vi "L_Cal_XYZ_Coordinate.vi"(9 "distance":dbl, 10 "vertical":dbl, 11 "azimuth":dbl) -> (1 "z":dbl, 2 "y":dbl, 3 "x":dbl)   [LabVIEW 2019]
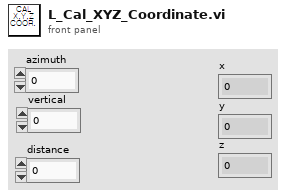
[diagram p1: front panel]
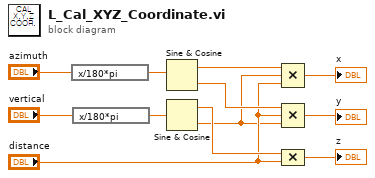
[diagram p0: block diagram]
diagram:
  n1 = expression code="x/180*pi"("azimuth") -> (w10:dbl)
  n2 = expression code="x/180*pi"("vertical") -> (w9:dbl)
  n3 = Sine & Cosine(0:w10) -> (1:w8:dbl, 2:w6:dbl)
  n4 = Sine & Cosine(0:w9) -> (1:w3:dbl, 2:w1:dbl)
  n5 = Compound Arithmetic op=MULTIPLY(w8, w1, "distance") -> (→"x":dbl)
  n6 = Compound Arithmetic op=MULTIPLY(w6, "distance", w1) -> (→"y":dbl)
  n7 = Compound Arithmetic op=MULTIPLY(w3, "distance") -> (→"z":dbl)
